vi "verify readout rate.vi"(8 "error in (no error)":errorcluster, 11 "Sim_Ixon_Ultra in":refnum<class "Sim_Ixon_Ultra.lvclass">) -> (0 "error out":errorcluster, 3 "Sim_Ixon_Ultra out":refnum<class "Sim_Ixon_Ultra.lvclass">)   [LabVIEW 2018, in "Sim_Ixon_Ultra.lvclass"]
uses:
  Sim_Ixon_Ultra.lvclass
  C:/Users/Denis/Desktop/S4ACS/S4ACS/Sim_CCD/Sim_CCD.lvclass
  Sim_CCD/Sim_CCD.lvclass
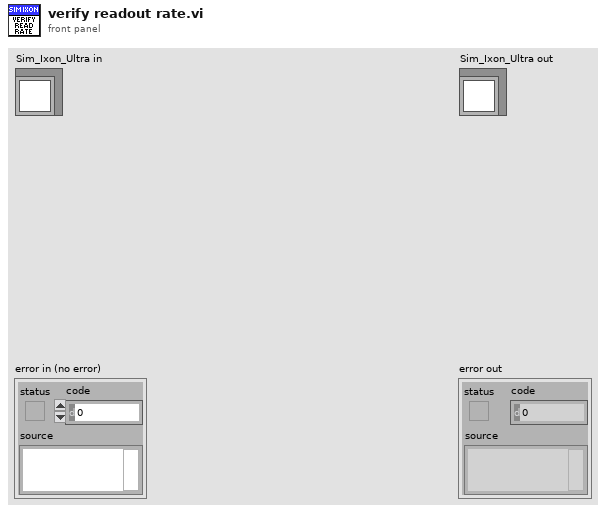
[diagram p1: front panel]
types:
  T1 = cluster{"PREAMP":u16, "READOUT_RATE":u16, "VERTICAL_SHIFT_SPEED":u16, "READ_MODE":u16, "VERTICAL_CLOCK_VOLTAGE":u16, "ACQUISITION_MODE":u16, "AD_CHANNEL":u16, "SHUTTER_TTL":u16, "SHUTTER_OPENING_TIME":u16, "SHUTTER_CLOSING_TIME":u16, "SHUTTER_MODE":u16, "TRIGGER_MODE":u16, "VBIN":u16, "INITIAL_LINE":u16, "INITIAL_COLUMN":u16, "FINAL_LINE":u16, "FINAL_COLUMN":u16, "HBIN":u16}
  T2 = cluster{"EM_MODE":u16, "EM_GAIN":u16, "FRAME_TRANSFER":bool}
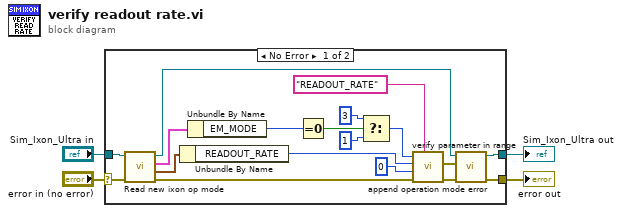
[diagram p0: block diagram]
diagram:
  n1 = case shown="No Error" "error in (no error)" {
    selector: "error in (no error)" -> [w21 w24]
    tunnel: [w5 w24] -> w3
    tunnel: [w6 w23] -> w1
    tunnel: "Sim_Ixon_Ultra in" -> [w22 w23]
    frame No Error {
      n2 = call-dynamic "Read new ixon op mode.vi"("error in (no error)"=w21, "Sim_Ixon_Ultra in"=w22) -> ("error out"=w8:errorcluster, "new operation mode"=w19:T1, "new ixon op mode"=w20:T2, "Sim_Ixon_Ultra out"=w7:refnum<class "Sim_Ixon_Ultra.lvclass">)  [unwired: 6 in]
      n3 = Unbundle By Name(w19) -> ("READOUT_RATE"=w12:u16)
      n4 = Unbundle By Name(w20) -> ("EM_MODE"=w18:u16)
      n5 = Equal To 0?(x=w18) -> (x = 0?=w17:bool)
      n6 = Select(t=3, s=w17, f=1) -> (s? t:f=w13:i32)
      n7 = call "verify parameter in range.vi"("parameter name"="READOUT_RATE", "error in (no error)"=w8, "lower limit"=0, "value"=w12, "upper limit"=w13) -> ("error out"=w9:errorcluster, "verific error"=w10:errorcluster)  [unwired: 5 in]
      n8 = call "append operation mode error.vi"("error in (no error)"=w9, "error"=w10, "Simulated_CCD_Camera in"=w7) -> ("error out"=w5:errorcluster, "Simulated_CCD_Camera out"=w6:refnum<class "Sim_Ixon_Ultra.lvclass">)  [unwired: 7 in]
    }
    frame Error {
    }
  }
  "error out" <- w3
  "Sim_Ixon_Ultra out" <- w1
